vi "HFRR ADV v011 new software.vi"() -> ()   [LabVIEW 2025] (continued)
            n2044 = Bundle "Bundle"(w1946, w2031) -> (w1965:cluster{dbl[], dbl[]})  [unwired: 1 in]
            n2045 = Bundle "Bundle"(w1977, w1973) -> (w1979:cluster{dbl[], dbl[]})  [unwired: 1 in]
            n2046 = Bundle "Bundle"(w1942, w1941) -> (w1949:cluster{dbl[], dbl[]})  [unwired: 1 in]
            n2047 = Bundle "Bundle"(w1975, w1971) -> (w1981:cluster{dbl[], dbl[]})  [unwired: 1 in]
            n2048 = Bundle "Bundle"(w1942, w1975) -> (w2085:cluster{dbl[], dbl[]})  [unwired: 1 in]
            n2049 = Bundle "Bundle"(w1942, w1971) -> (w2009:cluster{dbl[], dbl[]})  [unwired: 1 in]
            n2050 = Bundle "Bundle"(w1942, w2030) -> (w2095:cluster{dbl[], dbl[]})  [unwired: 1 in]
            n2051 = Bundle "Bundle"(w1942, w2025) -> (w2033:cluster{dbl[], dbl[]})  [unwired: 1 in]
            n2052 = Bundle "Bundle"(w1942, w2056) -> (w2080:cluster{dbl[], dbl[]})  [unwired: 1 in]
            n2053 = Bundle "Bundle"(w1976, w1972) -> (w1980:cluster{dbl[], dbl[]})  [unwired: 1 in]
            n2054 = Bundle "Bundle"(w1944, w1943) -> (w1950:cluster{dbl[], dbl[]})  [unwired: 1 in]
            n2055 = Bundle "Bundle"(w1944, w1976) -> (w2087:cluster{dbl[], dbl[]})  [unwired: 1 in]
            n2056 = Bundle "Bundle"(w1944, w1972) -> (w2010:cluster{dbl[], dbl[]})  [unwired: 1 in]
            n2057 = Bundle "Bundle"(w1944, w2026) -> (w2034:cluster{dbl[], dbl[]})  [unwired: 1 in]
            n2058 = Bundle "Bundle"(w1944, w2028) -> (w2096:cluster{dbl[], dbl[]})  [unwired: 1 in]
            n2059 = Bundle "Bundle"(w1944, w2065) -> (w2078:cluster{dbl[], dbl[]})  [unwired: 1 in]
            n2060 = Bundle "Bundle"(w1974, w1970) -> (w1982:cluster{dbl[], dbl[]})  [unwired: 1 in]
            n2061 = Bundle "Bundle"(w1940, w1939) -> (w1948:cluster{dbl[], dbl[]})  [unwired: 1 in]
            n2062 = Bundle "Bundle"(w1940, w1974) -> (w2086:cluster{dbl[], dbl[]})  [unwired: 1 in]
            n2063 = Bundle "Bundle"(w1940, w1970) -> (w2008:cluster{dbl[], dbl[]})  [unwired: 1 in]
            n2064 = Bundle "Bundle"(w1940, w2024) -> (w2032:cluster{dbl[], dbl[]})  [unwired: 1 in]
            n2065 = Bundle "Bundle"(w1940, w2029) -> (w2094:cluster{dbl[], dbl[]})  [unwired: 1 in]
            n2066 = Bundle "Bundle"(w1940, w2047) -> (w2079:cluster{dbl[], dbl[]})  [unwired: 1 in]
            n2067 = call-poly <vilib>:"Mean.vi"("X"=w2027) -> ("mean"=→"CP1":dbl)  [unwired: 1 out]
            n2068 = call-poly <vilib>:"Mean.vi"("X"=w1968) -> ("mean"=→"КОФ2 3":dbl)  [unwired: 1 out]
            n2069 = call-poly <vilib>:"Mean.vi"("X"=w2026) -> ("mean"=→"CP2":dbl)  [unwired: 1 out]
            n2070 = call-poly <vilib>:"Mean.vi"("X"=w2028) -> ("mean"=→"КОФ2":dbl)  [unwired: 1 out]
            n2071 = call-poly <vilib>:"Mean.vi"("X"=w1966) -> ("mean"=→"КОФ2 5":dbl)  [unwired: 1 out]
            n2072 = call-poly <vilib>:"Mean.vi"("X"=w2024) -> ("mean"=→"CP4":dbl)  [unwired: 1 out]
            n2073 = call-poly <vilib>:"Mean.vi"("X"=w2029) -> ("mean"=→"КОФ4":dbl)  [unwired: 1 out]
            n2074 = Bundle "Bundle"(w1946, w1973) -> (w1937:cluster{dbl[], dbl[]})  [unwired: 1 in]
            n2075 = Bundle "Bundle"(w1946, w2027) -> (w1960:cluster{dbl[], dbl[]})  [unwired: 1 in]
            n2076 = Build Array "Build Array"(w1937, w1960) -> (w1963:cluster{dbl[], dbl[]}[])
            "XY Graph 17" <- w1963
            n2077 = Build Array "Build Array"(w1951, w1950, w1949, w1948) -> (→"Frequency ( Hz )":cluster{dbl[], dbl[]}[])
            n2078 = Build Array "Build Array"(w1979, w1980, w1981, w1982) -> (→"Air Temp ( °C ) vs Humidity ( % RH )":cluster{dbl[], dbl[]}[])
            n2079 = Build Array "Build Array"(w1964, w2087, w2085, w2086) -> (→"Air Temperature  ( °C )":cluster{dbl[], dbl[]}[])
            n2080 = Build Array "Build Array"(w1937, w2010, w2009, w2008) -> (→"Humidity ( %RH )":cluster{dbl[], dbl[]}[])
            n2081 = Build Array "Build Array"(w1965, w2096, w2095, w2094) -> (→"Coefficient Of Friction":cluster{dbl[], dbl[]}[])
            n2082 = Build Array "Build Array"(w1960, w2034, w2033, w2032) -> (→"Sample Temperature ( °C )":cluster{dbl[], dbl[]}[])
            n2083 = Build Array "Build Array"(w1938, w2078, w2080, w2079) -> (→"XY Graph 13":cluster{dbl[], dbl[]}[])
            n2084 = Bundle "Bundle"(w1946, w1969) -> (w1991:cluster{dbl[], dbl[]})  [unwired: 1 in]
            n2085 = Bundle "Bundle"(w1942, w1967) -> (w1989:cluster{dbl[], dbl[]})  [unwired: 1 in]
            n2086 = Bundle "Bundle"(w1944, w1968) -> (w1990:cluster{dbl[], dbl[]})  [unwired: 1 in]
            n2087 = Bundle "Bundle"(w1940, w1966) -> (w1988:cluster{dbl[], dbl[]})  [unwired: 1 in]
            n2088 = Build Array "Build Array"(w1991, w1990, w1989, w1988) -> (→"Stroke ( mm )":cluster{dbl[], dbl[]}[])
            n2089 = local write "XY Graph 16"(w1963) -> ()
          }
          frame #2 {
          }
          frame #3 {
            n2090 = local write "Numeric 8"(0 ("Numeric 8")) -> ()
            n2091 = local write "Numeric 11"(0 ("Numeric 11")) -> ()
            n2092 = local write "Numeric 12"(0 ("Numeric 12")) -> ()
            n2093 = local write "Numeric 13"(0 ("Numeric 13")) -> ()
            n2094 = property on="OPEN" class="Bool (strict)"("Visible"=TRUE) -> ()  [unwired: 2 in, 2 out]
            n2095 = local read "String Control 2"() -> (w2263:string)
            n2096 = local read "String Control 4"() -> (w2262:string)
            n2097 = local read "String Control 6"() -> (w2261:string)
            n2098 = local read "String Control 8"() -> (w2260:string)
            n2099 = Match Pattern(string=w2263, regular expression="Samples / cycle :- ") -> (after substring=w2277:string)  [unwired: 1 in, 3 out]
            n2100 = Match Pattern(string=w2263, regular expression="Frequency :- ") -> (after substring=w2296:string)  [unwired: 1 in, 3 out]
            n2101 = Match Pattern(string=w2262, regular expression="Samples / cycle :- ") -> (after substring=w2273:string)  [unwired: 1 in, 3 out]
            n2102 = Match Pattern(string=w2262, regular expression="Frequency :- ") -> (after substring=w2291:string)  [unwired: 1 in, 3 out]
            n2103 = Match Pattern(string=w2261, regular expression="Samples / cycle :- ") -> (after substring=w2269:string)  [unwired: 1 in, 3 out]
            n2104 = Match Pattern(string=w2261, regular expression="Frequency :- ") -> (after substring=w2286:string)  [unwired: 1 in, 3 out]
            n2105 = Match Pattern(string=w2260, regular expression="Samples / cycle :- ") -> (after substring=w2265:string)  [unwired: 1 in, 3 out]
            n2106 = Match Pattern(string=w2260, regular expression="Frequency :- ") -> (after substring=w2281:string)  [unwired: 1 in, 3 out]
            n2107 = String Subset(string=w2277, length (rest)=6 ("length (rest)")) -> (substring=w2279:string)  [unwired: 1 in]
            n2108 = String Subset(string=w2296, length (rest)=9 ("length (rest)")) -> (substring=w2298:string)  [unwired: 1 in]
            n2109 = String Subset(string=w2273, length (rest)=6 ("length (rest)")) -> (substring=w2275:string)  [unwired: 1 in]
            n2110 = String Subset(string=w2291, length (rest)=9 ("length (rest)")) -> (substring=w2293:string)  [unwired: 1 in]
            n2111 = String Subset(string=w2269, length (rest)=6 ("length (rest)")) -> (substring=w2271:string)  [unwired: 1 in]
            n2112 = String Subset(string=w2286, length (rest)=9 ("length (rest)")) -> (substring=w2288:string)  [unwired: 1 in]
            n2113 = String Subset(string=w2265, length (rest)=6 ("length (rest)")) -> (substring=w2267:string)  [unwired: 1 in]
            n2114 = String Subset(string=w2281, length (rest)=9 ("length (rest)")) -> (substring=w2283:string)  [unwired: 1 in]
            n2115 = Fract/Exp String To Number(string=w2279) -> (number=w2259:dbl)  [unwired: 3 in, 1 out]
            n2116 = Fract/Exp String To Number(string=w2298) -> (number=w2299:dbl)  [unwired: 3 in, 1 out]
            n2117 = Fract/Exp String To Number(string=w2275) -> (number=w2258:dbl)  [unwired: 3 in, 1 out]
            n2118 = Fract/Exp String To Number(string=w2293) -> (number=w2294:dbl)  [unwired: 3 in, 1 out]
            n2119 = Fract/Exp String To Number(string=w2271) -> (number=w2257:dbl)  [unwired: 3 in, 1 out]
            n2120 = Fract/Exp String To Number(string=w2288) -> (number=w2289:dbl)  [unwired: 3 in, 1 out]
            n2121 = Fract/Exp String To Number(string=w2267) -> (number=w2256:dbl)  [unwired: 3 in, 1 out]
            n2122 = Fract/Exp String To Number(string=w2283) -> (number=w2284:dbl)  [unwired: 3 in, 1 out]
            n2123 = local write "sample1"(w2259) -> ()
            n2124 = local write "freq1"(w2299) -> ()
            n2125 = local write "sample2"(w2258) -> ()
            n2126 = local write "freq2"(w2294) -> ()
            n2127 = local write "sample3"(w2257) -> ()
            n2128 = local write "freq3"(w2289) -> ()
            n2129 = local write "sample4"(w2256) -> ()
            n2130 = local write "freq 4"(w2284) -> ()
          }
        }
      }
    }
    n2131 = case shown="True" w1748 {
      selector: w1748 -> [_ w1876]
      frame False {
      }
      frame True {
        n2132 = Not(x=w1876) -> (.not. x?=w1872:bool)
        n2133 = local write "service 3"(w1872) -> ()
        n2134 = local write "OPEN 6"(w1872) -> ()
        n2135 = call <vilib>:"System Exec.vi"("wait until completion? (T)"=TRUE, "command line"="C:\\LAB-IQ\\Scar View.exe") -> ("error out"=→"error out 5":errorcluster)  [unwired: 6 in, 3 out]
      }
    }
    n2136 = case shown="\"Acquire\", Default" w1759 {
      frame "Acquire", Default {
        w2772 = 0.2 ("y")
        w2777 = 1.0 ("y")
        w2778 = 0.8 ("y")
        # "Elapsed time\ncof\nstroke\nAir temp\nTemp\nHumidity"
        n2137 = disable-structure shown="Disabled" {
          frame Disabled {
            n2138 = local read "Flag"() -> (w2795:dbl)
            n2139 = local read "RUN"() -> (w2792:bool)
            n2140 = Not(x=w2792) -> (.not. x?=w2791:bool)
            n2141 = Equal?(x=w2795, y=10.0) -> (x = y?=w2793:bool)
            n2142 = And(x=w2793, y=w2791) -> (x .and. y?=w2790:bool)
            n2143 = case shown="True" w2790 {
              frame False {
              }
              frame True {
                w2796 = FALSE ("Heater Button")
                n2144 = local write "Humidity"(w2796) -> ()
                n2145 = local write "Heater Button"(w2796) -> ()
              }
            }
          }
          frame Enabled {
          }
        }
        n2146 = disable-structure shown="Disabled" {
          frame Disabled {
            n2147 = case shown="True" {
              selector: _ -> [_ _]
              frame False {
              }
              frame True {
                w2887 = TRUE ("Heater")
                n2148 = local write "Humidity"(w2887) -> ()
                n2149 = local write "Heater Button"(w2887) -> ()
                n2150 = local read "TEST STANDARD"() -> (w2890:T3)
                n2151 = local read "TEST STANDARD"() -> (w2885:T3)
                n2152 = Equal?(x=w2890, y=enum16{"ASTM D6079", "ISO 12156", "Custom"}."ISO 12156" ("Test Standard")) -> (x = y?=w2888:bool)
                n2153 = Equal?(x=w2885, y=enum16{"ASTM D6079", "ISO 12156", "Custom"}."ASTM D6079" ("Test Standard")) -> (x = y?=w2884:bool)
                n2154 = case shown="True" w2888 {
                  frame False {
                  }
                  frame True {
                    n2155 = local write "Heater"(TRUE ("Heater")) -> ()
                    n2156 = local write "airtempflg"(FALSE ("airtempflg")) -> ()
                  }
                }
                n2157 = case shown="True" w2884 {
                  frame False {
                  }
                  frame True {
                    n2158 = local write "Heater"(FALSE ("Heater")) -> ()
                    n2159 = local write "airtempflg"(TRUE ("airtempflg")) -> ()
                  }
                }
              }
            }
          }
          frame Enabled {
          }
        }
        n2160 = stacked-sequence {
          frame #0 {
            n2161 = case shown="True" "RST FF" {
              frame False {
              }
              frame True {
                w2953 = 0.0 ("X Scale.Range:Maximum")
                n2162 = property on="Frictional Force ( N )" class="WFChart (strict)"("XScale.Maximum"=600.0 ("X Scale.Range:Maximum"), "XScale.Minimum"=w2953, "YScale.Maximum"=10.0 ("Y Scale.Range:Maximum"), "YScale.Minimum"=w2953) -> ()  [unwired: 2 in, 2 out]
              }
            }
          }
          frame #1 {
            n2163 = case shown="True" "RST TEMP" {
              frame False {
              }
              frame True {
                n2164 = property on="Temperature ( Deg C )" class="WFChart (strict)"("XScale.Minimum"=0.0 ("X Scale.Range:Minimum"), "XScale.Maximum"=600.0 ("X Scale.Range:Maximum"), "YScale.Minimum"=0.0 ("Y Scale.Range:Minimum"), "YScale.Maximum"=100.0 ("Y Scale.Range:Maximum")) -> ()  [unwired: 2 in, 2 out]
              }
            }
          }
          frame #2 {
            n2165 = case shown="True" "RSTCOF" {
              frame False {
              }
              frame True {
                n2166 = property on="Coefficient of Friction" class="WFChart (strict)"("XScale.Minimum"=0.0 ("X Scale.Range:Minimum"), "XScale.Maximum"=600.0 ("X Scale.Range:Maximum"), "YScale.Maximum"=1.0 ("X Scale.Range:Minimum"), "YScale.Minimum"=0.0 ("X Scale.Range:Minimum")) -> ()  [unwired: 2 in, 2 out]
              }
            }
          }
          frame #3 {
            n2167 = case shown="True" "RSTCOF 2" {
              frame False {
              }
              frame True {
                (unwired) 100.0 ("Y Scale.Range:Maximum")
                (unwired) 0.0 ("Y Scale.Range:Minimum")
                (unwired) 600.0 ("X Scale.Range:Maximum")
                (unwired) 0.0 ("X Scale.Range:Minimum")
              }
            }
          }
          frame #4 {
            n2168 = case shown="True" "RSTCOF 3" {
              frame False {
              }
              frame True {
                n2169 = property on="Electrical Contact Resistance ( % )" class="WFChart (strict)"("XScale.Minimum"=0.0 ("X Scale.Range:Minimum"), "XScale.Maximum"=600.0 ("X Scale.Range:Maximum"), "YScale.Minimum"=0.0 ("Y Scale.Range:Minimum"), "YScale.Maximum"=100.0 ("Y Scale.Range:Maximum")) -> ()  [unwired: 2 in, 2 out]
              }
            }
          }
        }
        n2170 = disable-structure shown="Disabled" {
          frame Disabled {
            n2171 = case shown="True" {
              selector: _ -> [_ _]
              frame False {
              }
              frame True {
                n2172 = local read "zflag 2"() -> (w2854:dbl)
                n2173 = local read "yflag"() -> (w2856:dbl)
                n2174 = Equal?(x=w2856, y=2.0 ("tflag")) -> (x = y?=w2858:bool)
                n2175 = Equal?(x=w2854, y=3.0 ("tflag")) -> (x = y?=w2857:bool)
                n2176 = And(x=w2858, y=w2857) -> (x .and. y?=w2852:bool)
                n2177 = case shown="True" w2852 {
                  frame False {
                  }
                  frame True {
                    w2883 = 0.0 ("zflag")
                    n2178 = local write "zflag"(w2883) -> ()
                    n2179 = local write "zflag 2"(w2883) -> ()
                    n2180 = Delete(path (use dialog)=path "C:/LAB-IQ-NXT/WO 2449 TT.sig" ("file path (dialog if empty)")) -> (deleted path=w2882:path)  [unwired: 4 in, 2 out]
                    n2181 = Delete(path (use dialog)=path "C:/LAB-IQ-NXT/WO 2449 TRH.sig" ("file path (dialog if empty)")) -> (deleted path=w2877:path)  [unwired: 4 in, 2 out]
                    n2182 = local read "SEN.RUN HRS"() -> (w2869:dbl)
                    n2183 = local read "SENSOR TIME"() -> (w2867:dbl)
                    n2184 = call <vilib>:"compatOverwrite.vi"("overwrite (F)"=TRUE) -> ("overwrite?"=w2859:T29)
                    n2185 = call <vilib>:"compatOverwrite.vi"("overwrite (F)"=TRUE) -> ("overwrite?"=w2863:T29)
                    n2186 = local read "Total No. of Tests"() -> (w2870:dbl)
                    n2187 = Add(x=w2867, y=w2869) -> (x+y=w2868:dbl)
                    "SEN.RUN HRS" <- w2868
                    n2188 = Open/Create/Replace File(file path (use dialog)=w2882, operation (0:open)=w2859) -> (refnum out=w2860:refnum<file>, error out=w2861:errorcluster)  [unwired: 4 in, 1 out]
                    n2189 = Open/Create/Replace File(file path (use dialog)=w2877, operation (0:open)=w2863) -> (refnum out=w2864:refnum<file>, error out=w2865:errorcluster)  [unwired: 4 in, 1 out]
                    n2190 = Deny Access(4:w2861, 6:T27."deny none" ("deny mode (2)"), 7:w2860) -> (3:w2881:refnum<file>)  [unwired: 1 out]
                    n2191 = Deny Access(4:w2865, 6:T27."deny none" ("deny mode (2)"), 7:w2864) -> (3:w2873:refnum<file>)  [unwired: 1 out]
                    n2192 = Number To Decimal String(number=w2870) -> (decimal integer string=w2878:string)  [unwired: 1 in]
                    n2193 = Number To Decimal String(number=w2868) -> (decimal integer string=w2874:string)  [unwired: 1 in]
                    n2194 = Write to Binary File(file (use dialog)=w2881, data=w2878, 5:FALSE ("prepend array or string size? (T)")) -> ()  [unwired: 3 in, 3 out]
                    n2195 = Write to Binary File(file (use dialog)=w2873, data=w2874, 5:FALSE ("prepend array or string size? (T)")) -> ()  [unwired: 3 in, 3 out]
                  }
                }
              }
            }
          }
          frame Enabled {
          }
        }
        n2196 = local read "RUN"() -> (w2781:bool)
        n2197 = local read "run replace"() -> (w2785:bool)
        n2198 = local read "run replace"() -> (w2784:bool)
        n2199 = case shown="True" w2781 {
          frame False {
            n2200 = local write "run replace"(FALSE ("run replace")) -> ()
          }
          frame True {
            "run replace" <- TRUE ("run replace")
          }
        }
        n2201 = local read "RUN"() -> (w2789:bool)
        n2202 = local read "Set Temp"() -> (w2751:dbl)
        n2203 = local read "SetTemp"() -> (w2753:dbl)
        n2204 = case shown="False" w2789 {
          tunnel: [FALSE ("TEST RUNNING") TRUE ("TEST RUNNING")] -> w2788
          frame False {
            w2972 = 0.0 ("Flag")
            n2205 = local write "Elapsed time"(0.0 ("elapsedtime")) -> ()
            n2206 = local write "Time Remaining"(w2972) -> ()
            n2207 = local write "Flag"(w2972) -> ()
            n2208 = local write "Remaining Time"(w2972) -> ()
          }
          frame True {
            n2209 = local write "Flag"(10.0 ("Flag")) -> ()
          }
        }
        n2210 = case shown="False" w2785 {
          frame False {
            n2211 = local read "zflag"() -> (→"zflag 2":dbl)
            n2212 = local write "yflag"(2.0 ("tflag")) -> ()
            n2213 = local write "FLAG 4"(0.0 ("FLAG")) -> ()
          }
          frame True {
            n2214 = local write "yflag"(1.0 ("tflag")) -> ()
            n2215 = local write "zflag"(3.0 ("zflag")) -> ()
          }
        }
        n2216 = local read "acq 2"() -> (w2783:bool)
        n2217 = local read "AIR TEMP"() -> (w2746:dbl)
        n2218 = local read "Amb temp"() -> (w2750:dbl)
        n2219 = case shown="True" "Save & Continue" {
          frame False {
          }
          frame True {
            "acq 2" <- TRUE ("acq 2")
          }
        }
        n2220 = local read "Set Rh"() -> (w2752:dbl)
        n2221 = Add(x=w2753, y=w2778) -> (x+y=w2779:dbl)
        n2222 = Subtract(x=w2753, y=w2778) -> (x-y=w2780:dbl)
        n2223 = Add(x=w2751, y=w2772) -> (x+y=w2773:dbl)
        n2224 = Subtract(x=w2751, y=w2772) -> (x-y=w2774:dbl)
        n2225 = And(x=w2783, y=w2784) -> (x .and. y?=w2782:bool)
        n2226 = Greater Or Equal?(x=w2746, y=15.0) -> (x >= y?=w2747:bool)
        "powstat" <- w2747
        n2227 = local read "Humidity ( %RH )"() -> (w2749:dbl)
        n2228 = case shown="True" "Save & Continue" {
          frame False {
          }
          frame True {
            n2229 = while {
              tunnel: "0123456789abcdefghijklmnopqrstuvwxyzABCDEFGHIJKLMNOPQRSTUVWXYZ" ("string 2") -> [w2943]
              shift-right: [w2941] -> w2936
              shift-left: "" -> [w2940]
              i -> [w2950]
              stop <- w2949 stop-if-true
              n2230 = Random Number (0-1)() -> (number: 0 to 1=w2944:dbl)
              n2231 = Multiply(x=w2944, y=62.0) -> (x*y=w2946:dbl)
              n2232 = Decrement(x="Length") -> (x-1=w2939:i16)
              n2233 = To Word Integer(number=w2946) -> (16bit integer=w2947:i16)
              n2234 = String Subset(string=w2943, offset (0)=w2947, length (rest)=1 ("length (rest)")) -> (substring=w2942:string)
              n2235 = Greater Or Equal?(x=w2950, y=w2939) -> (x >= y?=w2949:bool)
              n2236 = Concatenate Strings(w2942, w2940) -> (w2941:string)
            }
            n2237 = local write "UUID"(w2936) -> ()
          }
        }
        n2238 = In Range and Coerce(upper limit=w2779, x=w2750, lower limit=w2780) -> (In Range?=w2769:bool)  [unwired: 1 out]
        n2239 = Add(x=w2752, y=w2777) -> (x+y=w2776:dbl)
        n2240 = Subtract(x=w2752, y=w2777) -> (x-y=w2775:dbl)
        n2241 = local read "TEMP"() -> (w2748:dbl)
        n2242 = case shown="True" "Save & Continue" {
          frame False {
          }
          frame True {
            n2243 = local read "Operator ID"() -> (w3265:string)
            n2244 = local read "FILE"() -> (w3271:string)
            n2245 = String Length(string=w3271) -> (length=w3269:i32)
            n2246 = String Length(string=w3265) -> (length=w3266:i32)
            n2247 = Greater?(x=w3269, y=0) -> (0:w3268:bool)
            n2248 = Greater?(x=w3266, y=0) -> (0:w3264:bool)
            n2249 = And(x=w3268, y=w3264) -> (x .and. y?=w3263:bool)
            n2250 = case shown="True" w3263 {
              frame False {
                n2251 = stacked-sequence {
                  frame #0 {
                    n2252 = One Button Dialog(message="Please Enter a File Name and Operator ID to save data !", button name ("OK")="Ok") -> ()  [unwired: 1 out]
                  }
                  frame #1 {
                    n2253 = local write "Save & Continue"(FALSE ("OK Button")) -> ()
                  }
                }
                n2254 = local write "Save & Continue"(FALSE ("OK Button")) -> ()
              }
              frame True {
                n2255 = stacked-sequence {
                  frame #0 {
                    n2256 = local read "FILE"() -> (w3277:string)
                    n2257 = call "file check.vi"("file name in"=w3277) -> ("file name out"=w3276:string)  [unwired: 9 in, 1 out]
                    n2258 = call <vilib>:"Application Directory.vi"() -> ("Application Directory"=w3287:path)
                    n2259 = Build Path(base path=w3287, name or relative path="data") -> (appended path=w3286:path)
                    n2260 = call <vilib>:"Trim Whitespace.vi"("string"=w3276) -> ("trimmed string"=w3284:string)  [unwired: 1 in]
                    n2261 = call <vilib>:"Trim Whitespace.vi"("string"=w3276) -> ("trimmed string"=w3285:string)  [unwired: 1 in]
                    n2262 = List Folder(path=w3286) -> (folder names=w3282:string[])  [unwired: 3 in, 3 out]
                    n2263 = Match Pattern(string=w3284, regular expression="_(") -> (before substring=w3281:string)  [unwired: 1 in, 3 out]
                    n2264 = for {
                      tunnel: w3282 -> [w3296] mode=indexing
                      tunnel: w3281 -> [w3294]
                      shift-right: [w3292] -> w3279
                      shift-left: bool[] [] -> [w3293]
                      n2265 = Match Pattern(string=w3296, regular expression="_(") -> (before substring=w3295:string)  [unwired: 1 in, 3 out]
                      n2266 = Equal?(x=w3295, y=w3294) -> (x = y?=w3291:bool)
                      n2267 = case shown="True" w3291 {
                        tunnel: w3291 -> [_ w3299]
                        tunnel: w3293 -> [w3298 w3301]
                        tunnel: [w3298 w3300] -> w3292
                        frame False {
                        }
                        frame True {
                          n2268 = Insert Into Array(array=w3301, new element=w3299) -> (w3300:bool[])  [unwired: 1 in]
                        }
                      }
                    }
                    n2269 = Equal?(x=w3282, y=w3281) -> (x = y?=w3290:bool[])
                    n2270 = Or Array Elements(Boolean array=w3290) -> (logical OR=w3289:bool)
                    n2271 = Array Size(array=w3279) -> (size(s)=w3278:i32)
                    n2272 = case shown="True" w3289 {
                      tunnel: w3285 -> [_ w3309]
                      tunnel: w3278 -> [_ w3302]
                      frame False {
                      }
                      frame True {
                        n2273 = Number To Decimal String(number=w3302) -> (decimal integer string=w3305:string)  [unwired: 1 in]
                        n2274 = Search/Split String(string=w3309, search string/char (-)="_(" ("regular expression")) -> (substring before match=w3307:string)  [unwired: 1 in, 2 out]
                        n2275 = Concatenate Strings(w3307, "_(" ("regular expression"), w3305, ")" ("regular expression")) -> (w3303:string)
                        n2276 = local write "FILE"(w3303) -> ()
                      }
                    }
                  }
                  frame #1 {
                    w3311 = 0.0
                    w3324 = cluster{"y":dbl, dbl, "y":dbl}[] [] ("History Data")
                    w3325 = FALSE ("Heater Button")
                    (unwired) ")!" ("string")
                    (unwired) ")" ("string")
                    w3323 = dbl[] [] ("History Data")
                    w3329 = "\r"
                    # "C:\\WinDucom\\Data\\"
                    # "C:\\LAB-IQ-NXT\\data"
                    n2277 = local write "Humidity ( %RH )"(w3311) -> ()
                    n2278 = local write "Frequency ( Hz )"(w3311) -> ()
                    n2279 = local write "Stroke 3"(w3311) -> ()
                    n2280 = local write "speedop"(0.0 ("PIDclk 2")) -> ()
                    n2281 = local write "Set Temp 2"(65.0 ("Set Temp 2")) -> ()
                    n2282 = local write "AIR TEMP"(w3311) -> ()
                    n2283 = local write "clk"(0.0 ("clk")) -> ()
                    n2284 = local write "Stroke 4"(w3311) -> ()
                    n2285 = local write "COF 2"(w3311) -> ()
                    n2286 = local write "TEMP"(w3311) -> ()
                    n2287 = local write "ecr 3"(w3311) -> ()
                    n2288 = local write "FF 3"(w3311) -> ()
                    n2289 = local write "FF 2"(w3311) -> ()
                    n2290 = property on="Humidity ( %RH )" class="WFChart (strict)"("History Data"=w3323) -> ()  [unwired: 2 in, 2 out]
                    n2291 = property on="Coefficient of Friction" class="WFChart (strict)"("History Data"=w3323) -> ()  [unwired: 2 in, 2 out]
                    n2292 = property on="Coefficient of Friction" class="WFChart (strict)"("History Data"=w3323) -> ()  [unwired: 2 in, 2 out]
                    n2293 = property on="Frictional Force ( N )" class="WFChart (strict)"("History Data"=w3323) -> ()  [unwired: 2 in, 2 out]
                    n2294 = property on="Electrical Contact Resistance ( % )" class="WFChart (strict)"("History Data"=w3323) -> ()  [unwired: 2 in, 2 out]
                    n2295 = property on="Electrical Contact Resistance ( % )" class="WFChart (strict)"("History Data"=w3323) -> ()  [unwired: 2 in, 2 out]
                    n2296 = property on="Temperature ( Deg C )" class="WFChart (strict)"("History Data"=w3323) -> ()  [unwired: 2 in, 2 out]
                    n2297 = property on="Frictional Force ( N )" class="WFChart (strict)"("History Data"=w3323) -> ()  [unwired: 2 in, 2 out]
                    n2298 = property on="Coefficient of Friction" class="WFChart (strict)"("History Data"=w3323) -> ()  [unwired: 2 in, 2 out]
                    n2299 = property on="Frictional Force ( N )" class="WFChart (strict)"("History Data"=w3323) -> ()  [unwired: 2 in, 2 out]
                    n2300 = property on="Electrical Contact Resistance ( % )" class="WFChart (strict)"("History Data"=w3323) -> ()  [unwired: 2 in, 2 out]
                    n2301 = property on="Temperature ( Deg C )" class="WFChart (strict)"("History Data"=w3323) -> ()  [unwired: 2 in, 2 out]
                    n2302 = property on="Humidity ( %RH )" class="WFChart (strict)"("History Data"=w3323) -> ()  [unwired: 2 in, 2 out]
                    n2303 = property on="Stroke ( mm )" class="WFChart (strict)"("History Data"=w3324) -> ()  [unwired: 2 in, 2 out]
                    n2304 = property on="Stroke ( mm )" class="WFChart (strict)"("History Data"=w3324) -> ()  [unwired: 2 in, 2 out]
                    n2305 = local write "Humidity"(w3325) -> ()
                    n2306 = local write "Heater Button"(w3325) -> ()
                    n2307 = local read "FILE"() -> (w3319:string)
                    n2308 = disable-structure shown="Enabled" {
                      disable-tunnel: [w3364 _] -> w3310
                      frame Enabled {
                        n2309 = local read "NORMAL LOAD"() -> (w3364:dbl)
                      }
                      frame Disabled {
                      }
                    }
                    n2310 = call "file check.vi"("file name in"=w3319) -> ("error out"=w3322:errorcluster, "file name out"=w3316:string)  [unwired: 9 in]
                    n2311 = call "FILE PATH CREATION.vi"("error in"=w3322, "FILE NAME :"=w3316) -> ("FILE OUT"=w3315:path)  [unwired: 8 in, 1 out]
                    n2312 = Concatenate Strings(w3316, ".dgf" ("Substring")) -> (w3321:string)
                    n2313 = Concatenate Strings(w3316, ".duf" ("Substring")) -> (w3317:string)
                    n2314 = Multiply(x=w3310, y=1.0) -> (x*y=w3343:dbl)
                    n2315 = Build Path(base path=w3315, name or relative path=w3321) -> (appended path=w3314:path)
                    n2316 = Build Path(base path=w3315, name or relative path=w3317) -> (appended path=w3313:path)
                    n2317 = Number To Fractional String(number=w3343, width (-)=i16 5, precision (6)=i16 2) -> (F-format string=w3351:string)  [unwired: 1 in]
                    n2318 = local read "Fuel Discription :"() -> (w3339:string)
                    n2319 = local read "Batch Ref Num :"() -> (w3327:string)
                    n2320 = Get Date/Time String(date format (0)=enum16{"short", "long", "abbreviated"}."short") -> (date string=w3362:string, time string=w3359:string)  [unwired: 2 in]
                    n2321 = local read "Remarks :"() -> (w3338:string)
                    n2322 = Concatenate Strings("Load :- " ("Substring"), w3351, " grams ," ("Substring")) -> (w3350:string)
                    n2323 = local read "String 41"() -> (w3330:string)
                    n2324 = Concatenate Strings(w3339) -> (w3340:string)
                    n2325 = Concatenate Strings(w3327) -> (w3326:string)
                    n2326 = Concatenate Strings("tested by") -> (w3334:string)
                    n2327 = Concatenate Strings("(" ("Substring"), w3362, ")" ("Substring"), w3359) -> (w3332:string)
                    "concatenated string" <- w3332
                    n2328 = Concatenate Strings(w3338, "," ("string")) -> (w3337:string)
                    n2329 = Concatenate Strings("  TIME;      COF;       STROKE;     AIR TEMP;  TEMP;  HUMIDITY;  ECR; PID-OUT; FREQUENCY" ("Substring"), "\r") -> (w3346:string)
                    n2330 = Concatenate Strings(w3330, w3329, "Fuel Discription :-" ("Substring"), w3340, w3329, w3350, w3329, "Batch Ref Num :-" ("Substring"), w3326, w3329, " Remarks :- " ("Substring"), w3337, w3329, " Date :- " ("Substring"), w3332, w3329, "Tested By :-" ("Substring"), w3334) -> (w3344:string)
                    "REMARKS" <- w3344
                    n2331 = call <vilib>:"Write Characters To File.vi"("append to file? (new file:F)"=FALSE, "character string"=w3346, "file path (dialog if empty)"=w3314) -> ()  [unwired: 2 in, 1 out]
                    n2332 = call <vilib>:"Write Characters To File.vi"("append to file? (new file:F)"=FALSE, "character string"=w3344, "file path (dialog if empty)"=w3313) -> ()  [unwired: 2 in, 1 out]
                  }
                  frame #2 {
                    n2333 = local write "Cycles elapsed"(0 ("Cycles elapsed")) -> ()
                    n2334 = local write "cyclecount"(0 ("cyclecount")) -> ()
                    n2335 = local write "Save & Continue"(FALSE ("OK")) -> ()
                    n2336 = local write "autostrtflg"(TRUE ("autostrtflg")) -> ()
                    n2337 = local write "Save"(FALSE ("Save")) -> ()
                    n2338 = Get Date/Time In Seconds() -> (seconds since 1Jan1904=w3369:timestamp)
                    n2339 = To Double Precision Float(number=w3369) -> (double precision float=w3368:dbl)
                    n2340 = local write "acq timer"(w3368) -> ()
                    n2341 = One Button Dialog(message="Please ensure sample is mounted properly and machine is ready in all aspects for testing !", button name ("OK")="Ok") -> ()  [unwired: 1 out]
                  }
                  frame #3 {
                    n2342 = stacked-sequence {
                      frame #0 {
                        n2343 = local write "Main Dashboard Buttons"(T1."Dashboard" ("Main Dashboard Buttons")) -> ()
                        n2344 = local write "Main Tab"(T2."Acquire" ("Main Tab")) -> ()
                      }
                      frame #1 {
                        n2345 = local write "EVENT LOG"("" ("EVENT LOG")) -> ()
                      }
                      frame #2 {
                        n2346 = Wait (ms)(milliseconds to wait=u32 50) -> ()  [unwired: 1 out]
                      }
                      frame #3 {
                        n2347 = disable-structure shown="Disabled" {
                          frame Disabled {
                            n2348 = local read "EVENT LOG"() -> (w3381:string)
                            n2349 = call "Event Log.vi"("Content"="Test Details", "EVENT LOG"=w3381) -> ("EVENT LOG"=w3380:string)  [unwired: 8 in, 1 out]
                            n2350 = local write "EVENT LOG"(w3380) -> ()
                          }
                          frame Enabled {
                          }
                        }
                      }
                      frame #4 {
                        n2351 = Wait (ms)(milliseconds to wait=u32 50) -> ()  [unwired: 1 out]
                      }
                      frame #5 {
                        n2352 = local read "FILE"() -> (w3383:string)
                        n2353 = Concatenate Strings("File Name :" ("Content"), w3383) -> (w3384:string)
                        n2354 = local read "EVENT LOG"() -> (w3387:string)
                        n2355 = call "Event Log.vi"("Content"=w3384, "EVENT LOG"=w3387) -> ("EVENT LOG"=w3386:string)  [unwired: 8 in, 1 out]
                        n2356 = local write "EVENT LOG"(w3386) -> ()
                      }
                      frame #6 {
                        n2357 = Wait (ms)(milliseconds to wait=u32 50) -> ()  [unwired: 1 out]
                      }
                      frame #7 {
                        n2358 = local read "Batch Ref Num :"() -> (w3389:string)
                        n2359 = Concatenate Strings("Batch Ref No :" ("Content"), w3389) -> (w3390:string)
                        n2360 = local read "EVENT LOG"() -> (w3393:string)
                        n2361 = call "Event Log.vi"("Content"=w3390, "EVENT LOG"=w3393) -> ("EVENT LOG"=w3392:string)  [unwired: 8 in, 1 out]
                        n2362 = local write "EVENT LOG"(w3392) -> ()
                      }
                      frame #8 {
                        n2363 = Wait (ms)(milliseconds to wait=u32 50) -> ()  [unwired: 1 out]
                      }
                      frame #9 {
                        n2364 = local read "tested by"() -> (w3395:string)
                        n2365 = Concatenate Strings("Tested By :" ("Content"), w3395) -> (w3396:string)
                        n2366 = local read "EVENT LOG"() -> (w3399:string)
                        n2367 = call "Event Log.vi"("Content"=w3396, "EVENT LOG"=w3399) -> ("EVENT LOG"=w3398:string)  [unwired: 8 in, 1 out]
                        n2368 = local write "EVENT LOG"(w3398) -> ()
                      }
                      frame #10 {
                        n2369 = Wait (ms)(milliseconds to wait=u32 50) -> ()  [unwired: 1 out]
                      }
                      frame #11 {
                        n2370 = local read "TEST STANDARD"() -> (w3402:T3)
                        n2371 = case shown="\"ASTM D6079\", Default" w3402 {
                          tunnel: ["ASTM D6079" "ISO 12156" "CEC F-096-A-06" "Custom"] -> w3401
                          frame "ASTM D6079", Default {
                          }
                          frame "ISO 12156" {
                          }
                          frame "CEC F-096-A-06" {
                          }
                          frame "Custom" {
                          }
                        }
                        n2372 = Concatenate Strings("Test Standard :" ("Content"), w3401) -> (w3403:string)
                        n2373 = local read "EVENT LOG"() -> (w3406:string)
                        n2374 = call "Event Log.vi"("Content"=w3403, "EVENT LOG"=w3406) -> ("EVENT LOG"=w3405:string)  [unwired: 8 in, 1 out]
                        n2375 = local write "EVENT LOG"(w3405) -> ()
                      }
                      frame #12 {
                        n2376 = Wait (ms)(milliseconds to wait=u32 50) -> ()  [unwired: 1 out]
                      }
                      frame #13 {
                        n2377 = local read "Fuel Discription :"() -> (w3412:string)
                        n2378 = Concatenate Strings("Fuel Description :" ("Content"), w3412) -> (w3413:string)
                        n2379 = local read "EVENT LOG"() -> (w3416:string)
                        n2380 = call "Event Log.vi"("Content"=w3413, "EVENT LOG"=w3416) -> ("EVENT LOG"=w3415:string)  [unwired: 8 in, 1 out]
                        n2381 = local write "EVENT LOG"(w3415) -> ()
                      }
                      frame #14 {
                        n2382 = Wait (ms)(milliseconds to wait=u32 50) -> ()  [unwired: 1 out]
                      }
                      frame #15 {
                        n2383 = local read "Remarks :"() -> (w3418:string)
                        n2384 = Concatenate Strings("Remarks :" ("Content"), w3418) -> (w3419:string)
                        n2385 = local read "EVENT LOG"() -> (w3422:string)
                        n2386 = call "Event Log.vi"("Content"=w3419, "EVENT LOG"=w3422) -> ("EVENT LOG"=w3421:string)  [unwired: 8 in, 1 out]
                        n2387 = local write "EVENT LOG"(w3421) -> ()
                      }
                      frame #16 {
                        n2388 = Wait (ms)(milliseconds to wait=u32 50) -> ()  [unwired: 1 out]
                      }
                      frame #17 {
                        n2389 = local read "Operator ID"() -> (w3424:string)
                        n2390 = Concatenate Strings("Operator ID :" ("Content"), w3424) -> (w3426:string)
                        n2391 = local read "EVENT LOG"() -> (w3428:string)
                        n2392 = call "Event Log.vi"("Content"=w3426, "EVENT LOG"=w3428) -> ("EVENT LOG"=w3427:string)  [unwired: 8 in, 1 out]
                        n2393 = local write "EVENT LOG"(w3427) -> ()
                      }
                      frame #18 {
                        n2394 = Wait (ms)(milliseconds to wait=u32 50) -> ()  [unwired: 1 out]
                      }
                      frame #19 {
                        n2395 = disable-structure shown="Disabled" {
                          frame Disabled {
                            n2396 = local read "EVENT LOG"() -> (w3432:string)
                            n2397 = call "Event Log.vi"("Content"="Test Parameter", "EVENT LOG"=w3432) -> ("EVENT LOG"=w3431:string)  [unwired: 8 in, 1 out]
                            n2398 = local write "EVENT LOG"(w3431) -> ()
                          }
                          frame Enabled {
                          }
                        }
                      }
                      frame #20 {
                        n2399 = Wait (ms)(milliseconds to wait=u32 50) -> ()  [unwired: 1 out]
                      }
                      frame #21 {
                        n2400 = local read "Set Hz"() -> (w3436:dbl)
                        n2401 = Number To Fractional String(number=w3436, precision (6)=i16 2) -> (F-format string=w3435:string)  [unwired: 2 in]
                        n2402 = Concatenate Strings("Set Frequency [Hz] :" ("Content"), w3435) -> (w3438:string)
                        n2403 = local read "EVENT LOG"() -> (w3440:string)
                        n2404 = call "Event Log.vi"("Content"=w3438, "EVENT LOG"=w3440) -> ("EVENT LOG"=w3439:string)  [unwired: 8 in, 1 out]
                        n2405 = local write "EVENT LOG"(w3439) -> ()
                      }
                      frame #22 {
                        n2406 = Wait (ms)(milliseconds to wait=u32 50) -> ()  [unwired: 1 out]
                      }
                      frame #23 {
                        n2407 = local read "NORMAL LOAD"() -> (w3443:dbl)
                        n2408 = Number To Fractional String(number=w3443, precision (6)=i16 2) -> (F-format string=w3444:string)  [unwired: 2 in]
                        n2409 = Concatenate Strings("Applied Load [grams] :" ("Content"), w3444) -> (w3446:string)
                        n2410 = local read "EVENT LOG"() -> (w3448:string)
                        n2411 = call "Event Log.vi"("Content"=w3446, "EVENT LOG"=w3448) -> ("EVENT LOG"=w3447:string)  [unwired: 8 in, 1 out]
                        n2412 = local write "EVENT LOG"(w3447) -> ()
                      }
                      frame #24 {
                        n2413 = Wait (ms)(milliseconds to wait=u32 50) -> ()  [unwired: 1 out]
                      }
                      frame #25 {
                        n2414 = local read "Set Strk"() -> (w3451:dbl)
                        n2415 = Number To Fractional String(number=w3451, precision (6)=i16 2) -> (F-format string=w3452:string)  [unwired: 2 in]
                        n2416 = Concatenate Strings("Set Stroke [mm] :" ("Content"), w3452) -> (w3454:string)
                        n2417 = local read "EVENT LOG"() -> (w3456:string)
                        n2418 = call "Event Log.vi"("Content"=w3454, "EVENT LOG"=w3456) -> ("EVENT LOG"=w3455:string)  [unwired: 8 in, 1 out]
                        n2419 = local write "EVENT LOG"(w3455) -> ()
                      }
                      frame #26 {
                        n2420 = Wait (ms)(milliseconds to wait=u32 50) -> ()  [unwired: 1 out]
                      }
                      frame #27 {
                        n2421 = local read "Set Temp"() -> (w3459:dbl)
                        n2422 = Number To Fractional String(number=w3459, precision (6)=i16 2) -> (F-format string=w3460:string)  [unwired: 2 in]
                        n2423 = Concatenate Strings("Set Temperature [deg C] :" ("Content"), w3460) -> (w3462:string)
                        n2424 = local read "EVENT LOG"() -> (w3464:string)
                        n2425 = call "Event Log.vi"("Content"=w3462, "EVENT LOG"=w3464) -> ("EVENT LOG"=w3463:string)  [unwired: 8 in, 1 out]
                        n2426 = local write "EVENT LOG"(w3463) -> ()
                      }
                      frame #28 {
                        n2427 = Wait (ms)(milliseconds to wait=u32 50) -> ()  [unwired: 1 out]
                      }
                      frame #29 {
                        n2428 = local read "Set Rh"() -> (w3467:dbl)
                        n2429 = Number To Fractional String(number=w3467, precision (6)=i16 2) -> (F-format string=w3468:string)  [unwired: 2 in]
                        n2430 = Concatenate Strings("Set Humidity [%RH] :" ("Content"), w3468) -> (w3470:string)
                        n2431 = local read "EVENT LOG"() -> (w3472:string)
                        n2432 = call "Event Log.vi"("Content"=w3470, "EVENT LOG"=w3472) -> ("EVENT LOG"=w3471:string)  [unwired: 8 in, 1 out]
                        n2433 = local write "EVENT LOG"(w3471) -> ()
                      }
                      frame #30 {
                        n2434 = Wait (ms)(milliseconds to wait=u32 50) -> ()  [unwired: 1 out]
                      }
                      frame #31 {
                        n2435 = local read "test time"() -> (w3475:dbl)
                        n2436 = Number To Fractional String(number=w3475, precision (6)=i16 1) -> (F-format string=w3476:string)  [unwired: 2 in]
                        n2437 = Concatenate Strings("Test Duration [mins] :" ("Content"), w3476) -> (w3478:string)
                        n2438 = local read "EVENT LOG"() -> (w3480:string)
                        n2439 = call "Event Log.vi"("Content"=w3478, "EVENT LOG"=w3480) -> ("EVENT LOG"=w3479:string)  [unwired: 8 in, 1 out]
                        n2440 = local write "EVENT LOG"(w3479) -> ()
                      }
                      frame #32 {
                        w3481 = dbl[] [] ("History Data")
                        w3482 = cluster{"y":dbl, dbl, "y":dbl}[] [] ("History Data")
                        w3483 = FALSE ("Visible")
                        n2441 = property on="Stroke ( mm )" class="WFChart (strict)"("History Data"=w3482) -> ()  [unwired: 2 in, 2 out]
                        n2442 = property on="Humidity ( %RH )" class="WFChart (strict)"("History Data"=w3481) -> ()  [unwired: 2 in, 2 out]
                        n2443 = property on="Temperature ( Deg C )" class="WFChart (strict)"("History Data"=w3481) -> ()  [unwired: 2 in, 2 out]
                        n2444 = property on="Electrical Contact Resistance ( % )" class="WFChart (strict)"("History Data"=w3481) -> ()  [unwired: 2 in, 2 out]
                        n2445 = property on="Coefficient of Friction" class="WFChart (strict)"("History Data"=w3481) -> ()  [unwired: 2 in, 2 out]
                        n2446 = property on="Frictional Force ( N )" class="WFChart (strict)"("History Data"=w3481) -> ()  [unwired: 2 in, 2 out]
                        n2447 = property on="Coefficient of Friction" class="WFChart (strict)"("History Data"=w3481) -> ()  [unwired: 2 in, 2 out]
                        n2448 = property on="Frictional Force ( N )" class="WFChart (strict)"("History Data"=w3481) -> ()  [unwired: 2 in, 2 out]
                        n2449 = property on="Electrical Contact Resistance ( % )" class="WFChart (strict)"("History Data"=w3481) -> ()  [unwired: 2 in, 2 out]
                        n2450 = property on="Humidity ( %RH )" class="WFChart (strict)"("History Data"=w3481) -> ()  [unwired: 2 in, 2 out]
                        n2451 = property on="Stroke ( mm )" class="WFChart (strict)"("History Data"=w3482) -> ()  [unwired: 2 in, 2 out]
                        n2452 = property on="Temperature ( Deg C )" class="WFChart (strict)"("History Data"=w3481) -> ()  [unwired: 2 in, 2 out]
                        n2453 = property on="Service Password Log" class="Str"("Visible"=w3483) -> ()  [unwired: 2 in, 2 out]
                        n2454 = property on="Password 3" class="Clust (strict)"("Visible"=w3483) -> ()  [unwired: 2 in, 2 out]
                      }
                    }
                    "TEST FILE NAM,E SAVED" <- TRUE ("TEST FILE NAM,E SAVED")
                  }
                }
              }
            }
          }
        }
        n2455 = case shown="True" w2782 {
          frame False {
            n2456 = local write "tfalg"(0.0 ("tfalg")) -> ()
          }
          frame True {
            n2457 = local read "tfalg"() -> (w2927:dbl)
            n2458 = Equal?(x=w2927, y=0.0) -> (x = y?=w2928:bool)
            n2459 = case shown="True" w2928 {
              frame False {
              }
              frame True {
                n2460 = local read "Total No. of Tests"() -> (w2931:dbl)
                n2461 = local write "tfalg"(1.0 ("tfalg")) -> ()
                n2462 = local write "acq 2"(FALSE ("acq 2")) -> ()
                n2463 = Wait (ms)(milliseconds to wait=u32 200) -> ()  [unwired: 1 out]
                n2464 = Increment(x=w2931) -> (x+1=w2930:dbl)
                n2465 = local write "Total No. of Tests"(w2930) -> ()
              }
            }
          }
        }
        n2466 = local write "Test \nStatus"(w2788) -> ()
        n2467 = local write "Save"(w2788) -> ()
        n2468 = local read "Main Tab"() -> (w2745:T2)
        n2469 = case shown="True" w2769 {
          tunnel: [FALSE ("RUN") TRUE ("RUN")] -> w2768
          tunnel: [_ 1] -> w2761
          frame False {
          }
          frame True {
          }
        }
        n2470 = In Range and Coerce(upper limit=w2776, x=w2749, lower limit=w2775) -> (In Range?=w2767:bool)  [unwired: 1 out]
        n2471 = In Range and Coerce(upper limit=w2773, x=w2748, lower limit=w2774) -> (In Range?=w2765:bool)  [unwired: 1 out]
        n2472 = case shown="True" w2781 {
          frame False {
            n2473 = local read "Rt 3"() -> (w2909:bool)
            n2474 = case shown="True" w2909 {
              frame False {
              }
              frame True {
                n2475 = local write "Rt 3"(FALSE ("Rt 3")) -> ()
                n2476 = local write "Json End Flg"(TRUE ("Upld AR 2")) -> ()
              }
            }
            "Rt" <- TRUE ("Rt")
            "Rt 2" <- FALSE ("Rt")
          }
          frame True {
            n2477 = local read "Rt"() -> (w2916:bool)
            n2478 = local write "Rt 2"(TRUE ("Rt 2")) -> ()
            n2479 = case shown="True" w2916 {
              frame False {
              }
              frame True {
                w2917 = TRUE ("Upld AR 2")
                n2480 = local write "Rt"(FALSE ("Rt")) -> ()
                n2481 = local write "Upld AR"(w2917) -> ()
                n2482 = local write "Json St Flg"(w2917) -> ()
              }
            }
            "Rt 3" <- TRUE ("Rt 3")
          }
        }
        n2483 = case shown="True" w2767 {
          tunnel: [FALSE ("RUN") TRUE ("RUN")] -> w2766
          tunnel: [_ 2] -> w2760
          frame False {
          }
          frame True {
          }
        }
        n2484 = case shown="True" w2765 {
          tunnel: [FALSE ("RUN") TRUE ("RUN")] -> w2764
          tunnel: [_ 3] -> w2759
          frame False {
          }
          frame True {
          }
        }
        n2485 = case shown="\"Acquire\"" w2745 {
          tunnel: w2747 -> [_ w2978]
          frame Default {
            w2977 = 0.0 ("output")
            n2486 = local write "PID-out"(w2977) -> ()
            n2487 = local write "Frequency ( Hz )"(w2977) -> ()
          }
          frame "Acquire" {
            n2488 = stacked-sequence {
              frame #0 {
                n2489 = local read "Auto Start Test"() -> (w2980:bool)
                n2490 = case shown="True" w2980 {
                  tunnel: "RUN" -> [w3001 w3004]
                  tunnel: [w3001 w3003] -> w2981
                  frame False {
                  }
                  frame True {
                    n2491 = local read "Auto Start Temp"() -> (w3002:bool)
                    n2492 = Or(x=w3004, y=w3002) -> (x .or. y?=w3003:bool)
                  }
                }
                n2493 = local read "clk"() -> (w3000:dbl)
                n2494 = local read "Save"() -> (w2996:bool)
                n2495 = Equal?(x=w3000, y=0.0) -> (x = y?=w2997:bool)
                n2496 = And(x=w2997, y=w2996) -> (x .and. y?=w2998:bool)
                n2497 = Not(x="Engage") -> (.not. x?=w2987:bool)
                n2498 = case shown="False" w2981 {
                  tunnel: [0.0 w3027] -> w2983
                  frame False {
                    (unwired) TRUE ("Visible")
                    n2499 = local read "Auto Start Test"() -> (w3008:bool)
                    n2500 = local write "Start Time"(TRUE ("Start Time")) -> ()
                    n2501 = property on="Stroke 2" class="DigNum (strict)"("Visible"=FALSE) -> ()  [unwired: 2 in, 2 out]
                    n2502 = case shown="False" w3008 {
                      frame False {
                        n2503 = property on="Heater Button" class="Bool (strict)"("DisabledEnum"=T17."Enabled" ("Disabled")) -> ()  [unwired: 2 in, 2 out]
                        n2504 = property on="Humidity" class="Bool (strict)"("DisabledEnum"=T17."Enabled" ("Disabled")) -> ()  [unwired: 2 in, 2 out]
                      }
                      frame True {
                      }
                    }
                    n2505 = case shown="False" "TestCompFlg" {
                      frame False {
                        n2506 = local read "StartFlg"() -> (w3016:bool)
                        n2507 = case shown="True" w3016 {
                          frame False {
                          }
                          frame True {
                            n2508 = stacked-sequence {
                              frame #0 {
                                n2509 = local read "EVENT LOG"() -> (w3020:string)
                                n2510 = call "Event Log.vi"("Content"="Test was interrupted", "EVENT LOG"=w3020) -> ("EVENT LOG"=w3021:string)  [unwired: 8 in, 1 out]
                                n2511 = local write "EVENT LOG"(w3021) -> ()
                                n2512 = property on="RUN" class="Bool (strict)"("Visible"=TRUE) -> ()  [unwired: 2 in, 2 out]
                                n2513 = property on="Auto Start Test" class="Bool (strict)"("Visible"=TRUE) -> ()  [unwired: 2 in, 2 out]
                              }
                              frame #1 {
                                w3023 = FALSE ("StartFlg")
                                n2514 = property on="Heater Button" class="Bool (strict)"("Val(Sgnl)"=FALSE ("Value (Signaling)")) -> ()  [unwired: 2 in, 2 out]
                                n2515 = local write "Heater Button"(w3023) -> ()
                                n2516 = local write "StartFlg"(w3023) -> ()
                                n2517 = local write "Humidity"(w3023) -> ()
                              }
                              frame #2 {
                                n2518 = local write "Command"("VC;0" ("Command")) -> ()
                              }
                              frame #3 {
                                n2519 = Wait (ms)(milliseconds to wait=u32 1500) -> ()  [unwired: 1 out]
                              }
                              frame #4 {
                                n2520 = local write "Command"("HE;0" ("Command")) -> ()
                              }
                            }
                          }
                        }
                      }
                      frame True {
                      }
                    }
                    n2521 = local write "String 14"("Test will autostart once parameters reach the set value." ("String 14")) -> ()
                  }
                  frame True {
                    (unwired) FALSE ("Visible")
                    n2522 = property on="Stroke 2" class="DigNum (strict)"("Visible"=TRUE) -> ()  [unwired: 2 in, 2 out]
                    n2523 = property on="STOP 2" class="Bool (strict)"("Disabled"=u8 2) -> ()  [unwired: 2 in, 2 out]
                    n2524 = local write "String 14"(" Running....." ("String 14")) -> ()
                    n2525 = property on="Heater Button" class="Bool (strict)"("DisabledEnum"=T17."Disabled and Grayed Out" ("Disabled")) -> ()  [unwired: 2 in, 2 out]
                    n2526 = property on="Humidity" class="Bool (strict)"("DisabledEnum"=T17."Disabled and Grayed Out" ("Disabled")) -> ()  [unwired: 2 in, 2 out]
                    n2527 = case shown="True" "Start Time" {
                      selector: "Start Time" -> [_ w3046]
                      frame False {
                      }
                      frame True {
                        n2528 = Not(x=w3046) -> (.not. x?=w3045:bool)
                        n2529 = local write "Start Time"(w3045) -> ()
                        n2530 = local read "EVENT LOG"() -> (w3047:string)
                        n2531 = call "Event Log.vi"("Content"="Test in progress", "EVENT LOG"=w3047) -> ("EVENT LOG"=w3049:string)  [unwired: 8 in, 1 out]
                        n2532 = local write "EVENT LOG"(w3049) -> ()
                      }
                    }
                    n2533 = disable-structure shown="Enabled" {
                      disable-tunnel: [w3038 w3044] -> w3027
                      frame Disabled {
                        n2534 = local read "Set Hz"() -> (w3041:dbl)
                        n2535 = call <vilib>:"Uniform White Noise Waveform.vi"() -> ("signal out"=w3040:waveform(dbl))  [unwired: 10 in, 1 out]
                        n2536 = Random Number (0-1)() -> (number: 0 to 1=w3037:dbl)
                        n2537 = Add(x=w3041, y=w3040) -> (x+y=w3039:waveform(dbl))
                        n2538 = Multiply(x=ext 0.01 ("y"), y=w3037) -> (x*y=w3035:ext)
                        n2539 = Multiply(x=w3039, y=w3035) -> (x*y=w3038:waveform(ext))
                      }
                      frame Enabled {
                        n2540 = call-poly <vilib>:"Random Number (Range).vi"("lower bound (0)"=49.89, "upper bound (100)"=50.8) -> ("number"=w3044:dbl)  [unwired: 9 in]
                      }
                    }
                    "StartFlg" <- TRUE ("StartFlg")
                  }
                }
                n2541 = case shown="True" w2998 {
                  frame False {
                  }
                  frame True {
                    n2542 = local write "clk"(10.0 ("clk")) -> ()
                    n2543 = Get Date/Time In Seconds() -> (seconds since 1Jan1904=w3052:timestamp)
                    n2544 = To Double Precision Float(number=w3052) -> (double precision float=w3050:dbl)
                    n2545 = local write "acq timer"(w3050) -> ()
                    n2546 = local write "act save time"(w3050) -> ()
                  }
                }
                n2547 = call "Elapsed Time"("Time Target (s)"="Countdown", "Reset"=w2987) -> ("Elapsed Time (s)"=w2992:dbl, "Time has Elapsed"=w2990:bool)  [unwired: 10 in, 6 out]
                "Countdown 2" <- w2992
                n2548 = Subtract(x=w2992, y=2.0) -> (x-y=w2995:dbl)
                n2549 = Less?(x=w2995, y="Countdown") -> (x < y?=w2993:bool)
                n2550 = And(x=w2993, y=w2990) -> (x .and. y?=w2989:bool)
                n2551 = case shown="True" w2989 {
                  frame False {
                  }
                  frame True {
                    (unwired) dbl[] [] ("History Data")
                    n2552 = local write "Engage"(FALSE ("Engage")) -> ()
                    n2553 = local write "RUN"(TRUE ("RUN")) -> ()
                    n2554 = local read "Humidity ( %RH )"() -> (→"Rh Before":dbl)
                  }
                }
                n2555 = local read "Test \nStatus"() -> (w2985:bool)
                n2556 = Select(t=w2983, s=w2985, f=0.0) -> (s? t:f=w2984:dbl)
                n2557 = local write "Frequency ( Hz )"(w2984) -> ()
              }
              frame #1 {
                w3075 = 1000000.0 ("x")
                # "HC;1/0\nST;VALUE"
                # "Elapsed time\ncof\nstroke\nAir temp\nTemp\nHumidity"
                # "acq timer\n\nact save time"
                # "convert to microseconds"
                n2558 = local read "COUNT"() -> (w3058:i32)
                n2559 = local read "Rate"() -> (w3071:dbl)
                n2560 = Divide(x=w3075, y=w3071) -> (x/y=w3076:dbl)
                n2561 = Greater Or Equal?(x=w3058, y=250) -> (x >= y?=w3057:bool)
                n2562 = Get Date/Time In Seconds() -> (seconds since 1Jan1904=w3078:timestamp)
                n2563 = case shown="True" w3057 {
                  frame False {
                    n2564 = local read "COUNT"() -> (w3079:i32)
                    n2565 = Increment(x=w3079) -> (x+1=w3080:i32)
                    n2566 = local write "COUNT"(w3080) -> ()
                  }
                  frame True {
                    n2567 = local write "COUNT"(0 ("COUNT")) -> ()
                  }
                }
                n2568 = local read "Samplingtime 2"() -> (w3056:dbl)
                n2569 = local read "act save time"() -> (w3073:dbl)
                n2570 = Divide(x=w3076, y=w3075) -> (x/y=w3074:dbl)
                n2571 = To Double Precision Float(number=w3078) -> (double precision float=w3067:dbl)
                n2572 = Add(x=w3073, y=w3056) -> (x+y=w3072:dbl)
                n2573 = local read "acq timer"() -> (w3077:dbl)
                n2574 = local read "COUNT"() -> (w3060:i32)
                n2575 = Greater Or Equal?(x=w3067, y=w3072) -> (x >= y?=w3055:bool)
                n2576 = Multiply(x=w3074, y=w3060) -> (x*y=w3066:dbl)
                n2577 = Subtract(x=w3067, y=w3077) -> (x-y=w3069:dbl)
                n2578 = local read "Save"() -> (w3070:bool)
                n2579 = Add(x=w3069, y=w3066) -> (x+y=w3053:dbl)
                "Elapsed time 3" <- w3053
                n2580 = And(x=w3055, y=w3070) -> (x .and. y?=w3068:bool)
                n2581 = Divide(x=w3053, y=60.0) -> (x/y=w3064:dbl)
                n2582 = local read "Test \nStatus"() -> (w3054:bool)
                n2583 = local read "clk"() -> (w3061:dbl)
                n2584 = Equal?(x=w3061, y=10.0) -> (x = y?=w3063:bool)
                n2585 = case shown="True" w3068 {
                  tunnel: w3067 -> [_ w3189]
                  tunnel: [FALSE ("Boolean 2") TRUE ("Boolean 2")] -> _
                  frame False {
                  }
                  frame True {
                    w3143 = ";" ("Substring")
                    # "Pid out/\nFreq response value"
                    n2586 = local write "act save time"(w3189) -> ()
                    n2587 = local read "FILE"() -> (w3137:string)
